vi "GB_Vref Test.vi"(11 "Board Selector":T1) -> (0 "Error Out":errorcluster[](array[cluster]), 3 "Voltage Readings":dbl[](array[numeric]))   [LabVIEW 2022 SP3]
uses:
  Serial Board Com/Board Select.ctl
  Serial Board Com/ADCSelector GB.ctl
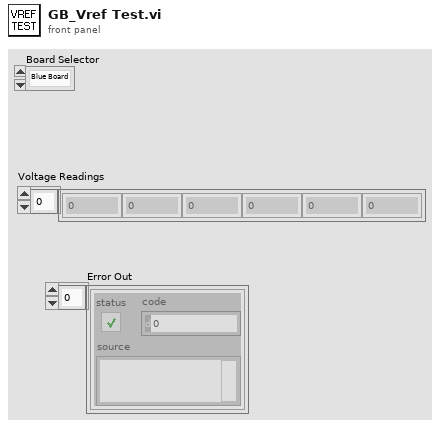
[diagram p1: front panel]
types:
  T1 = typedef "Board Select.ctl" = enum16{"Blue Board", "Green Board"}
  T2 = typedef "ADCSelector GB.ctl" = enum16{"INVA_ISENSE_U", "INVA_ISENSE_V", "INVA_ISENSE_W", "INVA_UDC", "INVA_TEMP", "HB_ISENSE", "AUX_ISENSE_U", "AUX_ISENSE_V", "AUX_ISENSE_W", "VLINE_AB", "VLINE_BC", "VLINE_CA", "REF_1P5V", "VSENSE_POS_24V", "VSENSE_POS_5V", "VSENSE_NEG_15V", "TEST_POINT", "INVB_ISENSE_U", "INVB_ISENSE_V", "INVB_ISENSE_W", "INVB_UDC", "INVB_TEMP", "HB_TEMP", "AUXA_TEMP", "AUXB_TEMP", "AUXC_TEMP", "VOUT_AB", "VOUT_BC", "VOUT_CA", "REF_2P5V", "VSENSE_POS_15V", "VSENSE_POS_3P3V", "NET_ANALYZER"}
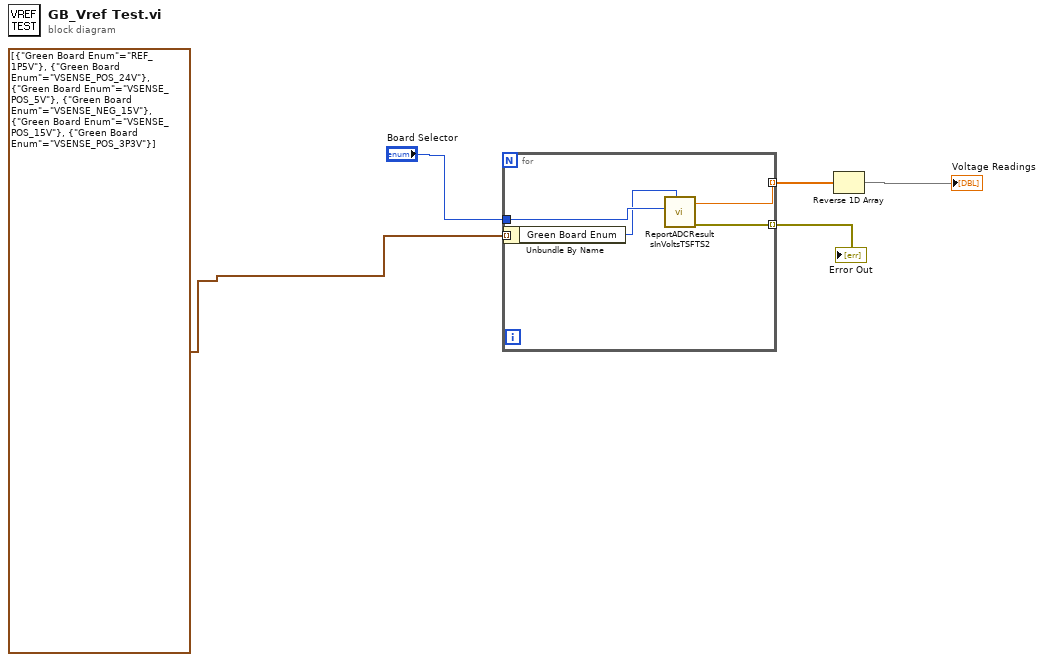
[diagram p0: block diagram]
diagram:
  n1 = for {
    tunnel: [w10] -> w5 mode=indexing
    tunnel: [w9] -> w3 mode=indexing
    tunnel: cluster{"Green Board Enum":T2}[] [{"Green Board Enum"=enum."REF_1P5V"}, {"Green Board Enum"=enum."VSENSE_POS_24V"}, {"Green Board Enum"=enum."VSENSE_POS_5V"}, {"Green Board Enum"=enum."VSENSE_NEG_15V"}, {"Green Board Enum"=enum."VSENSE_POS_15V"}, {"Green Board Enum"=enum."VSENSE_POS_3P3V"}] -> [w8] mode=indexing
    tunnel: "Board Selector" -> [w7]
    n2 = Unbundle By Name(w8) -> ("Green Board Enum"=w6:T2)
    n3 = call "ReportADCResultsInVoltsTSFTS2.vi"("Green Board Enum"=w6, "Board Selector"=w7) -> ("error out"=w9:errorcluster, "Result"=w10:dbl)  [unwired: 6 in, 2 out]
  }
  "Error Out" <- w3
  n4 = Reverse 1D Array(array=w5) -> (reversed array=→"Voltage Readings":dbl[])
